vi "Rem Read Handshake.vi"(11 "File Path Control":path) -> (0 "error out":errorcluster, 2 "string after HS bit":string, 3 "HS bit = 1":bool)   [LabVIEW 2014]
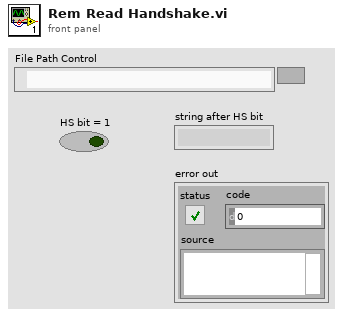
[diagram p1: front panel]
types:
  T1 = enum16{"open", "replace", "create", "open or create", "replace or create", "replace or create with confirmation"}
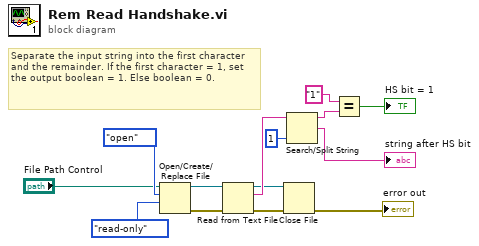
[diagram p0: block diagram]
diagram:
  # "Separate the input string into the first character\nand the remainder. If the first character = 1, set\nthe output boolean = 1. Else boolean = 0."
  n1 = Open/Create/Replace File(file path (use dialog)="File Path Control", operation (0:open)=T1."open", access (0:read/write)=enum16{"read/write", "read-only", "write-only"}."read-only") -> (refnum out=w4:refnum<file>, error out=w5:errorcluster)  [unwired: 3 in, 1 out]
  n2 = Read from Text File(file (use dialog)=w4, error in=w5) -> (refnum out=w7:refnum<file>, text=w9:string, error out=w6:errorcluster)  [unwired: 2 in, 1 out]
  n3 = Close File(refnum=w7, error in=w6) -> (error out=→"error out":errorcluster)  [unwired: 1 out]
  n4 = Search/Split String(string=w9, offset (0)=1) -> (substring before match=w13:string, match + rest of string=→"string after HS bit":string)  [unwired: 1 in, 1 out]
  n5 = Equal?(x="1", y=w13) -> (x = y?=→"HS bit = 1":bool)
